vi "niRFUtil LCAPI Copy 1D Array (1 I32, 5 DBL).vi"(0 "Source0 1D Array (I32)":i32[](array[numeric]), 1 "Source5 1D Array (DBL)":dbl[](array[numeric]) format="%.2f", 5 "Source1 1D Array (DBL)":dbl[](array[numeric]) format="%.2f", 7 "Source2 1D Array (DBL)":dbl[](array[numeric]) format="%.2f", 9 "Source3 1D Array (DBL)":dbl[](array[numeric]) format="%.2f", 11 "error in (no error)":errorcluster, 12 "Data Copy Descriptor":u64, 13 "Source4 1D Array (DBL)":dbl[](array[numeric]) format="%.2f") -> (2 "Source5 Out":dbl[](array[numeric]) format="%.2f", 3 "Source4 Out":dbl[](array[numeric]) format="%.2f", 4 "Source0 Out":i32[](array[numeric]), 6 "Source1 Out":dbl[](array[numeric]) format="%.2f", 8 "Source2 Out":dbl[](array[numeric]) format="%.2f", 10 "Source3 Out":dbl[](array[numeric]) format="%.2f", 15 "error out":errorcluster)   [LabVIEW 2015, in "niRFUtil.lvlib"]
uses:
  niRFUtil.lvlib
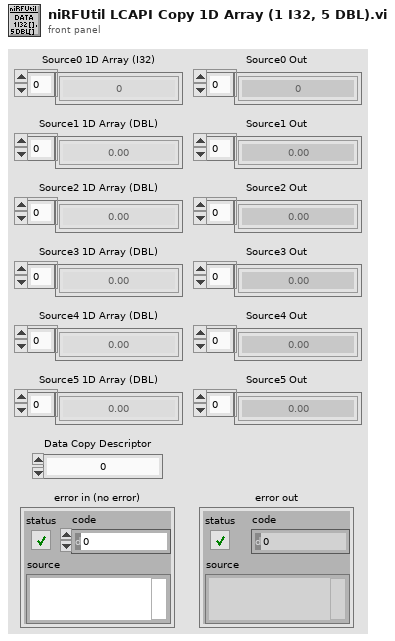
[diagram p1: front panel]
types:
  T1 = cluster{"status":bool, "return type":i32, "errorString":string}
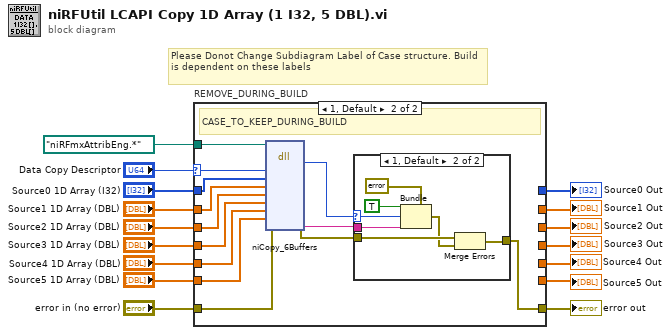
[diagram p0: block diagram]
diagram:
  # "Please Donot Change Subdiagram Label of Case structure. Build is dependent on these labels"
  n1 = case "REMOVE_DURING_BUILD" shown="1, Default" "Data Copy Descriptor" {
    selector: "Data Copy Descriptor" -> [_ w25]
    tunnel: [w23 w36] -> w16
    tunnel: "error in (no error)" -> [w23 w35]
    tunnel: "Source1 1D Array (DBL)" -> [w18 w34]
    tunnel: "Source2 1D Array (DBL)" -> [w19 w33]
    tunnel: "Source3 1D Array (DBL)" -> [w20 w32]
    tunnel: "Source5 1D Array (DBL)" -> [w22 w31]
    tunnel: "Source0 1D Array (I32)" -> [w17 w30]
    tunnel: "Source4 1D Array (DBL)" -> [w21 w29]
    tunnel: [w22 _] -> w7
    tunnel: [w21 _] -> w6
    tunnel: [w20 _] -> w5
    tunnel: [w19 _] -> w4
    tunnel: [w18 _] -> w3
    tunnel: [w17 _] -> w2
    tunnel: path "niRFmxAttribEng.*" ("path in") -> [_ w24]
    frame 0 {
      # "Development"
    }
    frame 1, Default {
      # "CASE_TO_KEEP_DURING_BUILD"
      n2 = dll-call lib="niRFmxAttribEng.*" fn="niCopy_6Buffers"(path in=w24, error in=w35, "dataCopyDescriptor"=w25, "source0"=w30, "source1"=w34, "source2"=w33, "source3"=w32, "source4"=w29, "source5"=w31) -> (error out=w26:errorcluster, "return type"=w28:i32, "errorString"=w27:string)  [unwired: 9 in, 1 out]
      n3 = case shown="1, Default" w28 {
        selector: w28 -> [_ w44]
        tunnel: w27 -> [_ w43]
        tunnel: w26 -> [w37 w41]
        tunnel: [w37 w42] -> w36
        frame 0 {
        }
        frame 1, Default {
          n4 = Bundle(cluster=T1 {"status"=FALSE, "return type"=0, "errorString"=""}, "status"=TRUE, "return type"=w44, "errorString"=w43) -> (w40:T1)
          n5 = Merge Errors(w41, w40) -> (w42:errorcluster)
        }
      }
    }
  }
  "error out" <- w16
  "Source0 Out" <- w2
  "Source1 Out" <- w3
  "Source2 Out" <- w4
  "Source3 Out" <- w5
  "Source5 Out" <- w7
  "Source4 Out" <- w6
